vi "Random Average.vi"() -> ()   [LabVIEW 2015]
panel:
  out "Waveform Chart":cluster{"number: 0 to 1":dbl, dbl}(graph)
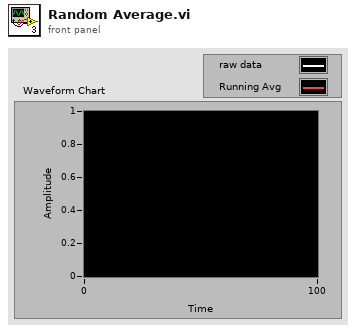
[diagram p1: front panel]
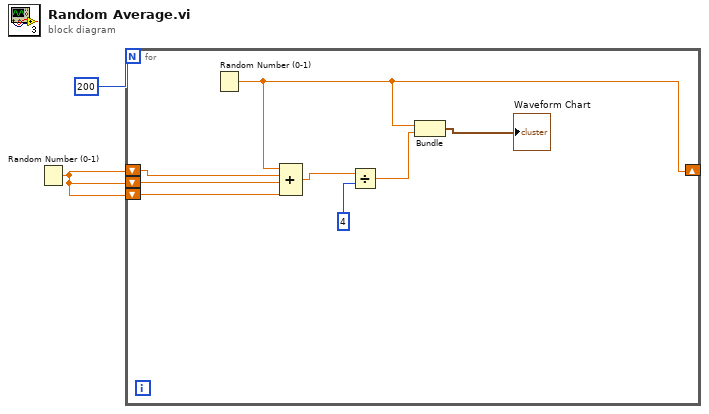
[diagram p0: block diagram]
diagram:
  n1 = Random Number (0-1)() -> (number: 0 to 1=w1:dbl)
  n2 = for {
    N: 200 -> [_]
    shift-right: [w5] -> _
    shift-left: w1 -> [w10]
    shift-left: w1 -> [w9]
    shift-left: w1 -> [w8]
    n3 = Random Number (0-1)() -> (number: 0 to 1=w5:dbl)
    n4 = Compound Arithmetic op=ADD(w5, w10, w9, w8) -> (w6:dbl)
    n5 = Divide(x=w6, y=4) -> (x/y=w4:dbl)
    n6 = Bundle("number: 0 to 1"=w5, w4) -> (→"Waveform Chart":cluster{"number: 0 to 1":dbl, dbl})  [unwired: 1 in]
  }
